vi "Enqueue Spectrum.vi"(8 "error in (no error)":errorcluster, 11 "Spectrum":cluster{"f0":dbl, "df":dbl, "magnitude":dbl[]}) -> (0 "error out":errorcluster)   [LabVIEW 2016]
uses:
  Utilities/Application Globals.vi
panel:
  out "overflow?":bool
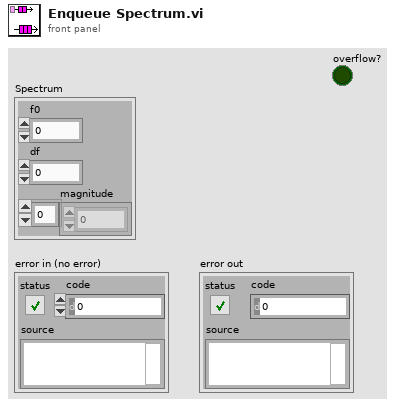
[diagram p1: front panel]
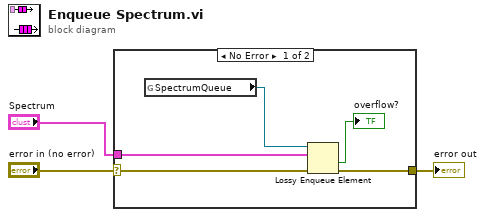
[diagram p0: block diagram]
diagram:
  n1 = case shown="No Error" "error in (no error)" {
    selector: "error in (no error)" -> [w6 w9]
    tunnel: "Spectrum" -> [w7 _]
    tunnel: [w5 w9] -> w3
    frame No Error {
      n2 = global read "Application Globals.vi" "SpectrumQueue"() -> (w8:refnum<queue>)
      n3 = Lossy Enqueue Element(queue=w8, element=w7, error in (no error)=w6) -> (overflow?=→"overflow?":bool, error out=w5:errorcluster)  [unwired: 2 out]
    }
    frame Error {
    }
  }
  "error out" <- w3
